vi "Untitled 1.vi"() -> ()   [LabVIEW 2023]
panel:
  in  "Saberi":bool
  in  "stop 2":bool
  in  "Podijeli":bool
  in  "Pomnozi":bool
  in  "Oduzmi":bool
  in  "Broj 2":dbl
  in  "Broj 1":dbl
  out "Rezultat":dbl
  in  "Pokreni":bool
  in  "Signal":enum16{"SINE", "COSINE"}(ring)
  out "Graph":dbl[](graph)
  out "XY Graph":cluster{dbl[], dbl[]}(graph)
  out "Waveform Graph 3":i32[](graph)
  out "Waveform Chart":i32[](graph)
  out "Waveform Graph 2":dynamicdata(graph)
  out "Waveform Graph":dynamicdata(graph)
  in  "stop":bool
  out "LED2":bool
  out "LED1":bool
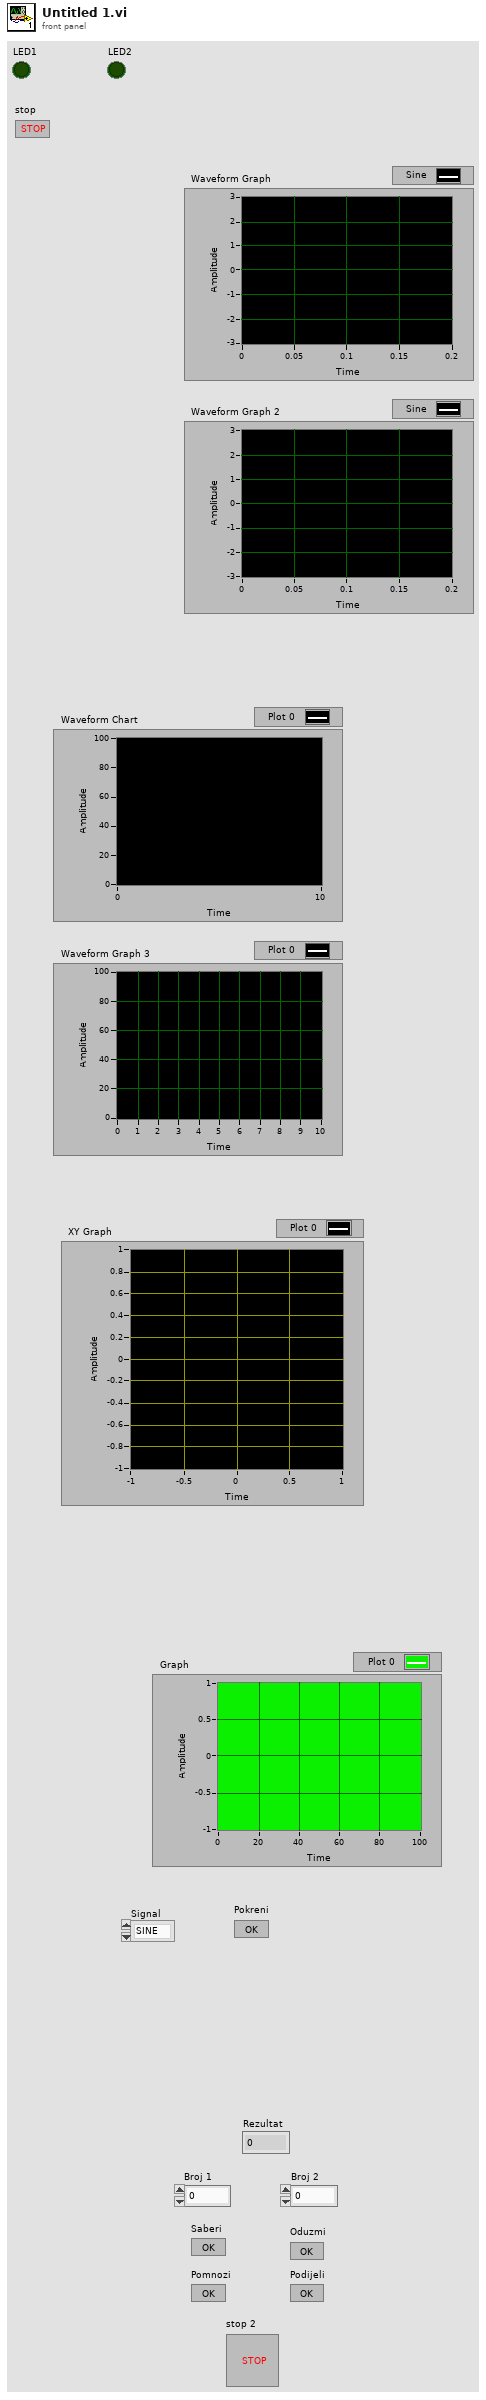
[diagram p1: front panel]
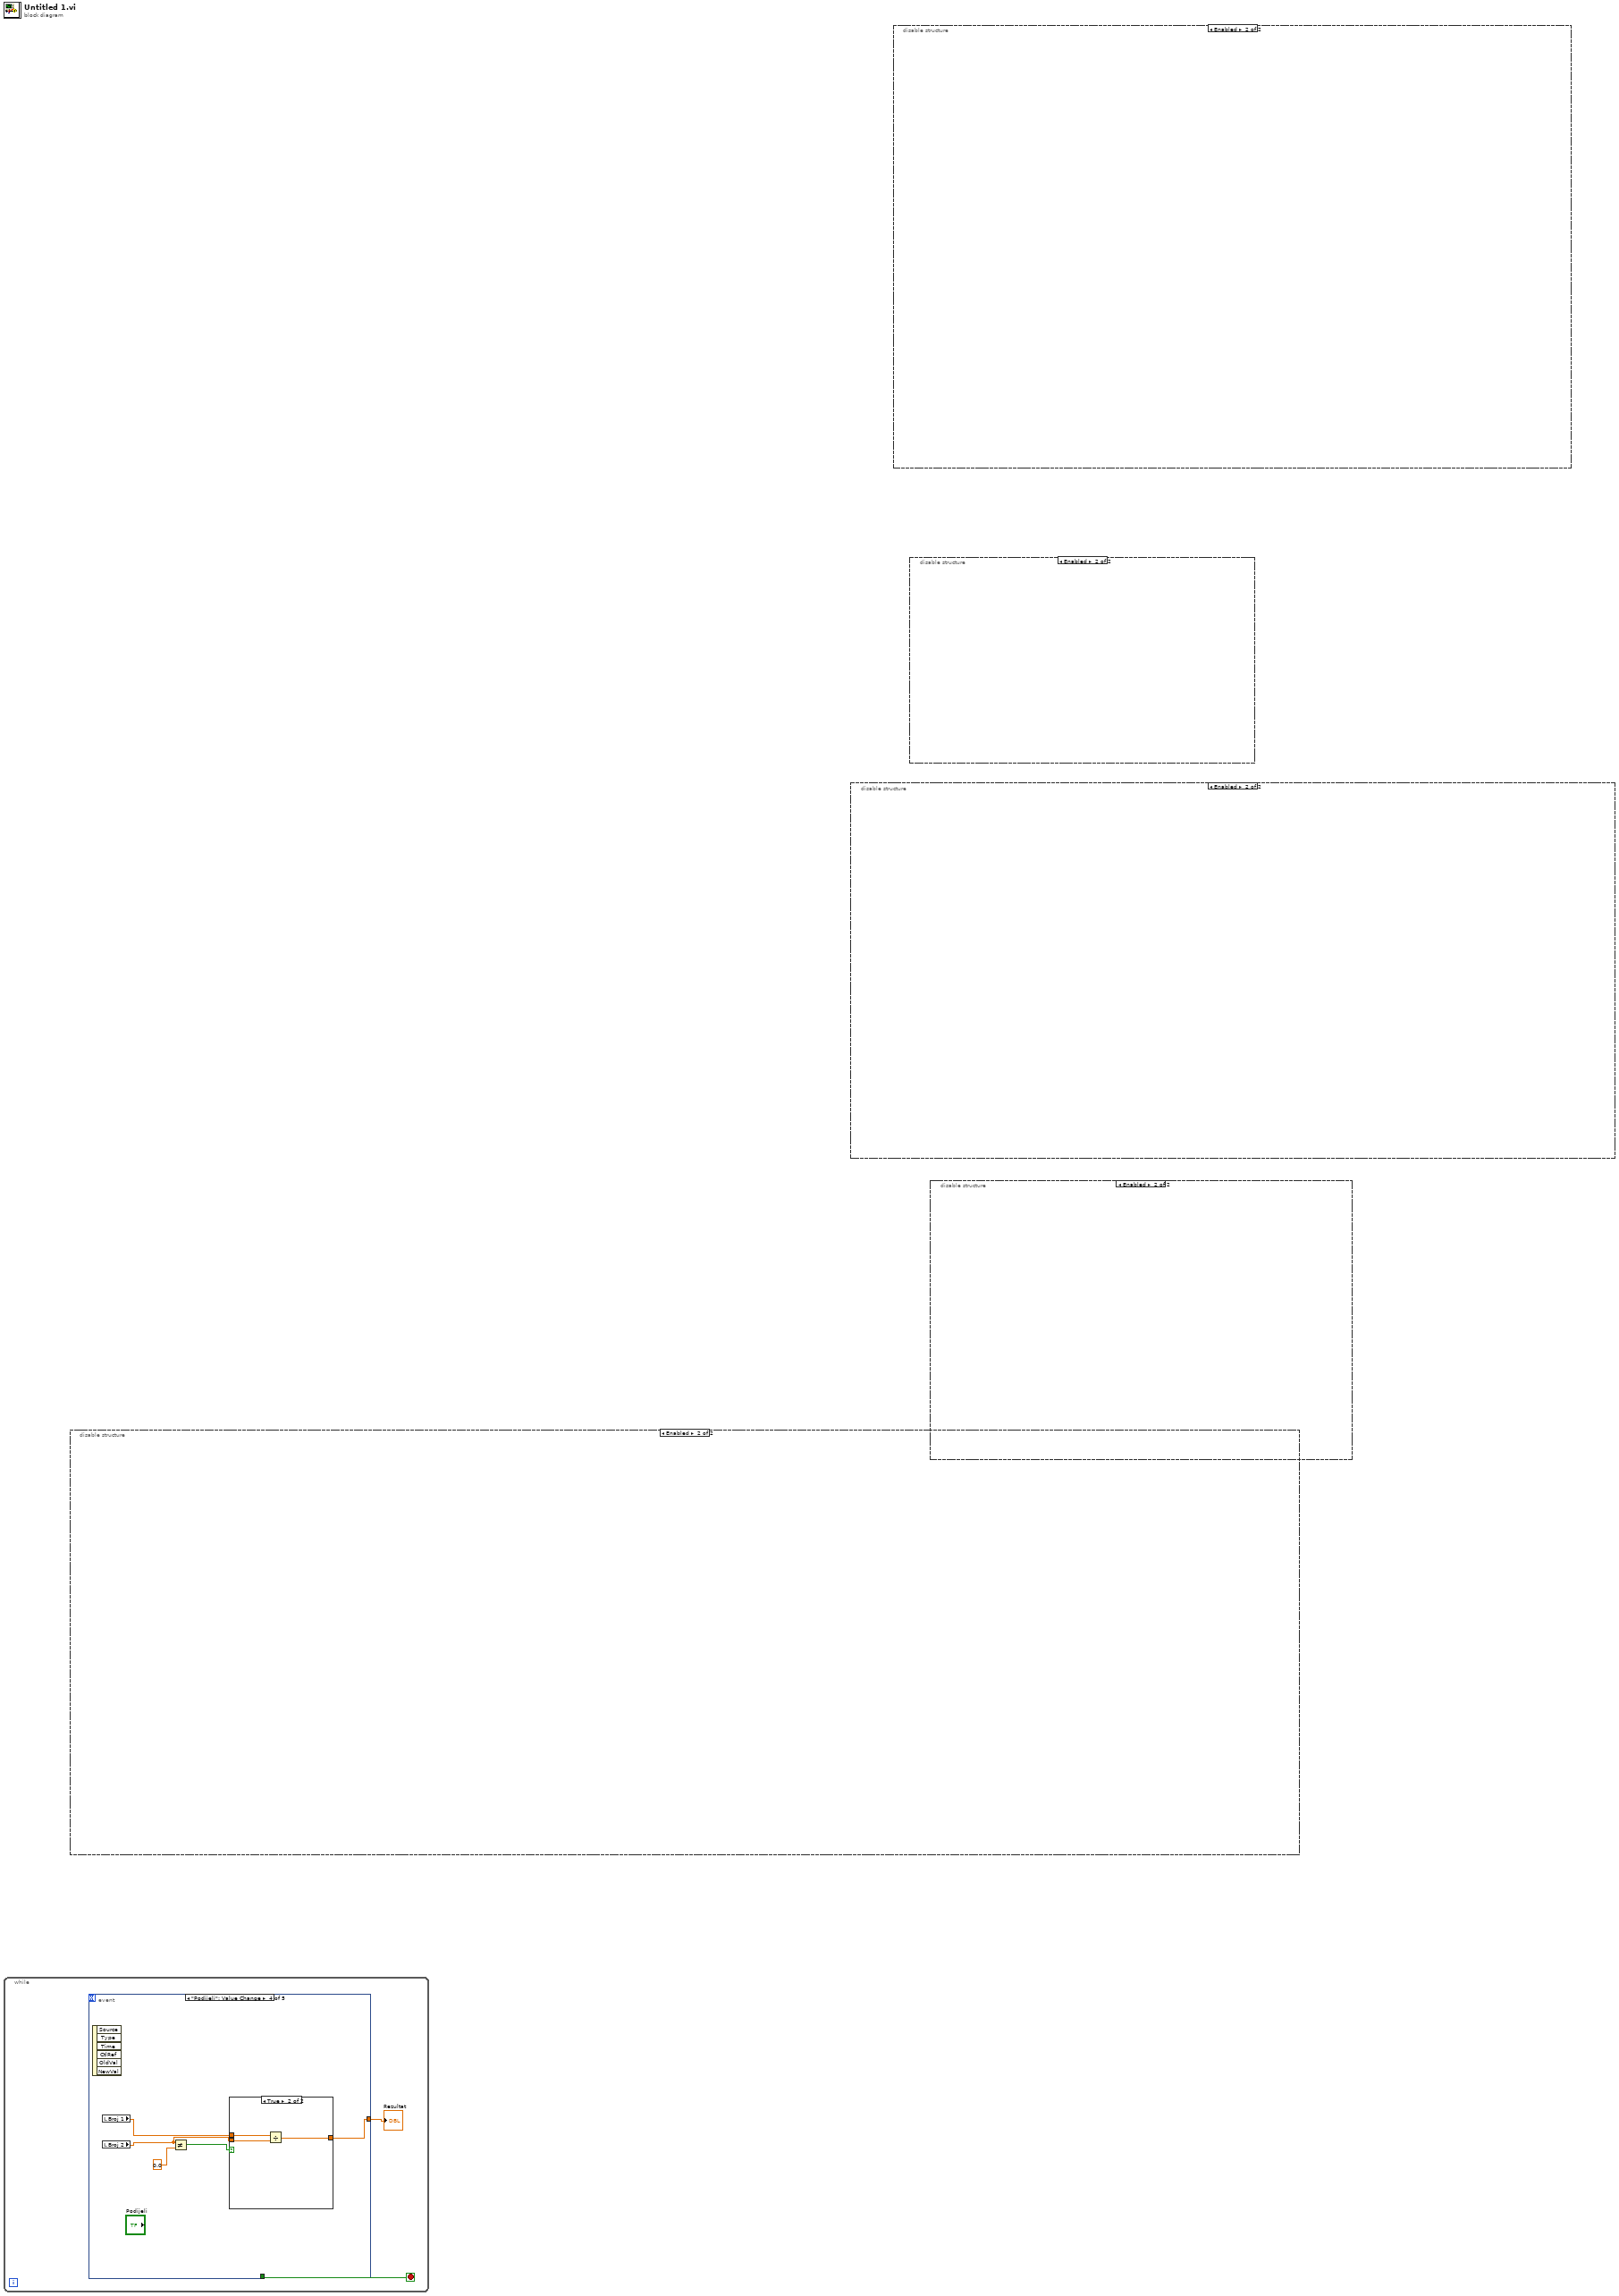
[diagram p0: block diagram]
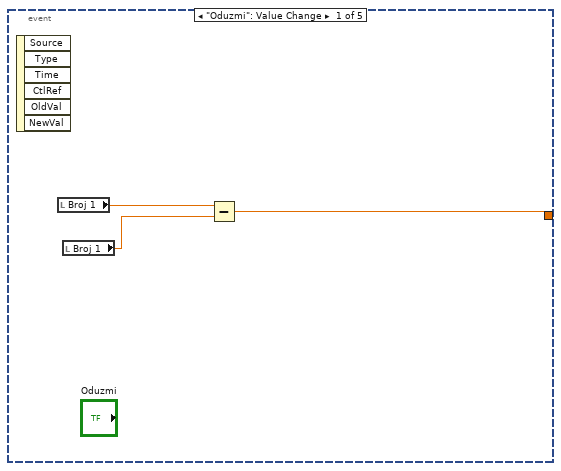
[diagram p2: hidden frame]
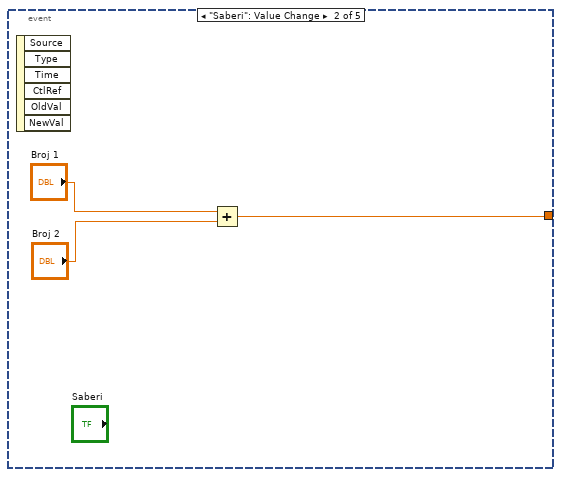
[diagram p3: hidden frame]
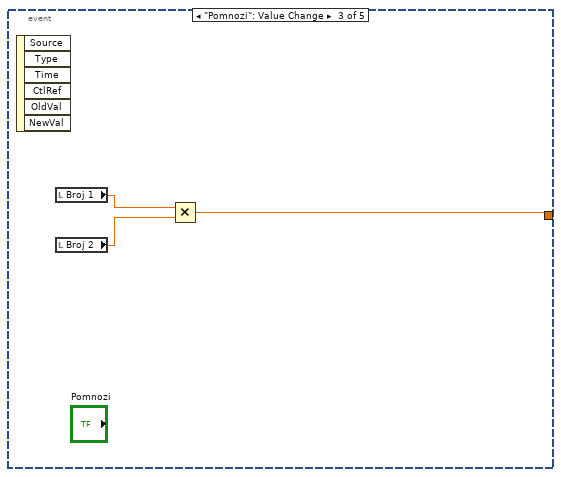
[diagram p4: hidden frame]
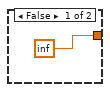
[diagram p5: hidden frame]
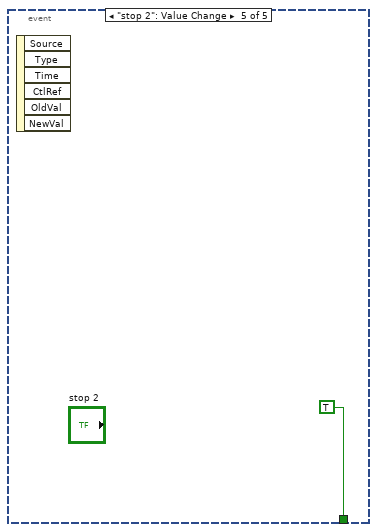
[diagram p6: hidden frame]
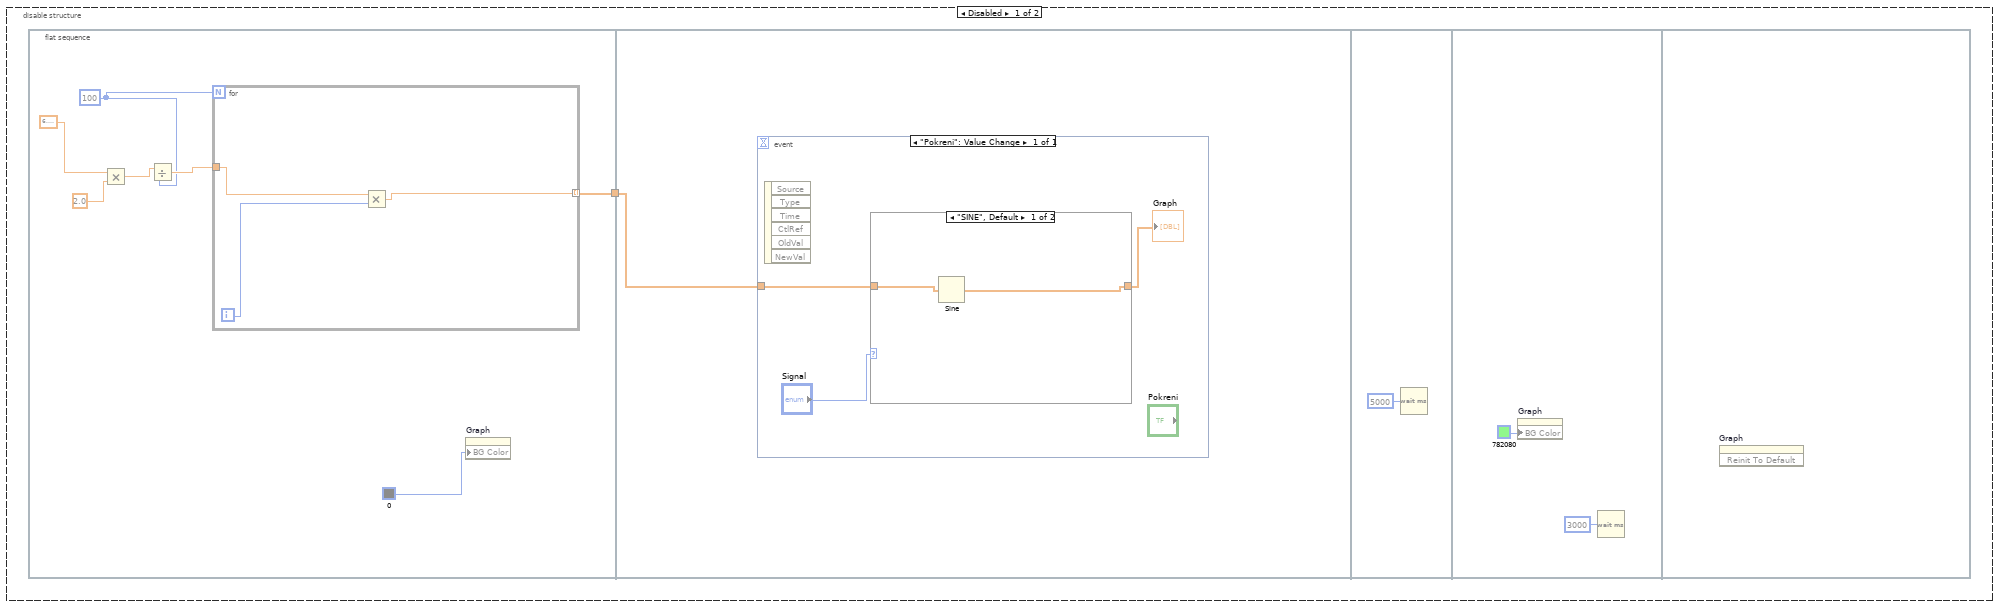
[diagram p7: hidden frame]
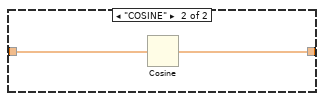
[diagram p8: hidden frame]
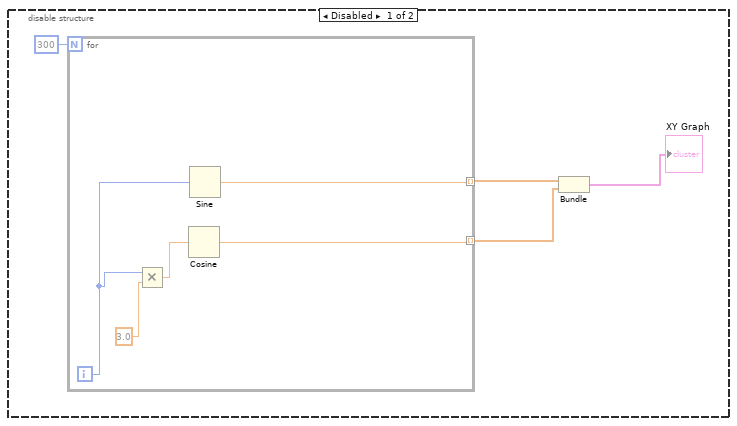
[diagram p9: hidden frame]
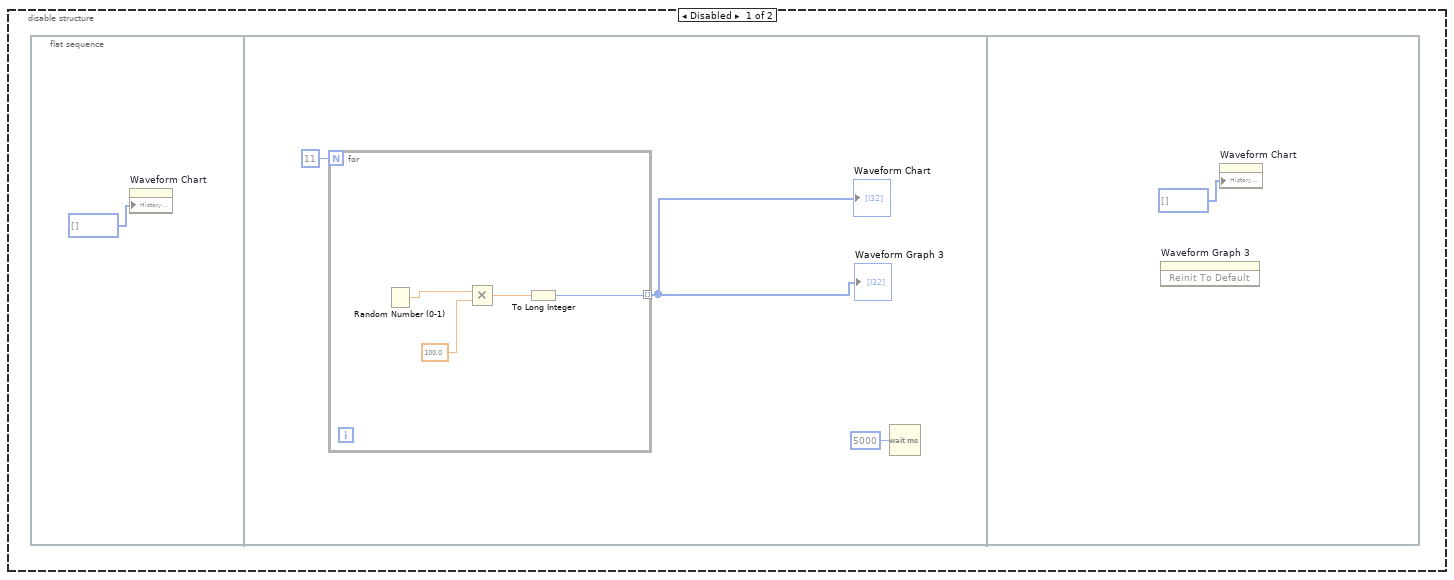
[diagram p10: hidden frame]
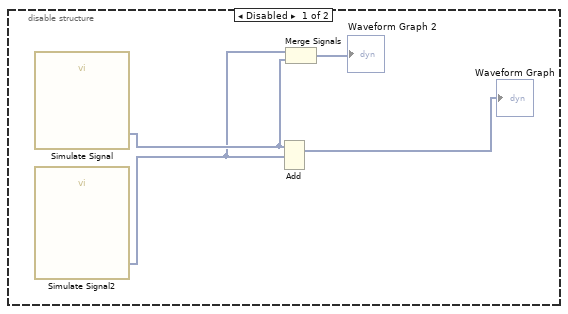
[diagram p11: hidden frame]
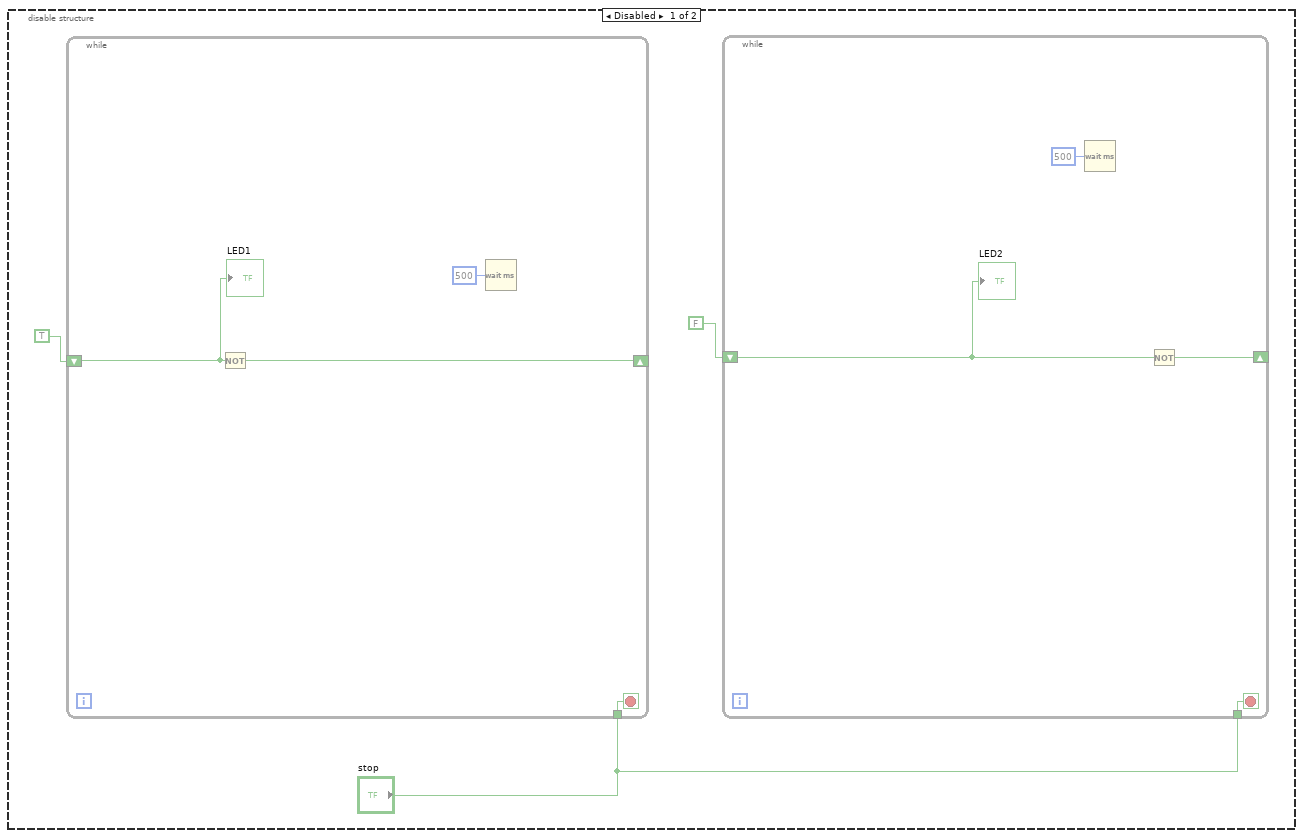
[diagram p12: hidden frame]
diagram:
  n1 = while {
    stop <- w2 stop-if-true
    n2 = event shown="[3] \"Podijeli\": Value Change" {
      selector: _ -> [_ _ _ _ _]
      dyn-events: _ -> [_ _ _ _ _]
      timeout: _ -> [_ _ _ _ _]
      tunnel: [w5 w8 w11 w14 _] -> w1
      tunnel: [_ _ _ _ TRUE] -> w2
      event "Oduzmi": Value Change {
        n3 = event-data() -> ()  [unwired: 1 in, 6 out]
        n4 = local read "Broj 1"() -> (w4:dbl)
        n5 = local read "Broj 1"() -> (w3:dbl)
        n6 = Subtract(x=w4, y=w3) -> (x-y=w5:dbl)
      }
      event "Saberi": Value Change {
        n7 = event-data() -> ()  [unwired: 1 in, 6 out]
        n8 = Add(x="Broj 1", y="Broj 2") -> (x+y=w8:dbl)
      }
      event "Pomnozi": Value Change {
        n9 = event-data() -> ()  [unwired: 1 in, 6 out]
        n10 = local read "Broj 1"() -> (w10:dbl)
        n11 = local read "Broj 2"() -> (w9:dbl)
        n12 = Multiply(x=w10, y=w9) -> (x*y=w11:dbl)
      }
      event "Podijeli": Value Change {
        n13 = event-data() -> ()  [unwired: 1 in, 6 out]
        n14 = local read "Broj 1"() -> (w13:dbl)
        n15 = local read "Broj 2"() -> (w12:dbl)
        n16 = Not Equal?(x=w12, y=0.0) -> (x != y?=w15:bool)
        n17 = case shown="True" w15 {
          tunnel: [inf w20] -> w14
          tunnel: w13 -> [_ w19]
          tunnel: w12 -> [_ w18]
          frame False {
          }
          frame True {
            n18 = Divide(x=w19, y=w18) -> (x/y=w20:dbl)
          }
        }
      }
      event "stop 2": Value Change {
        n19 = event-data() -> ()  [unwired: 1 in, 6 out]
      }
    }
    "Rezultat" <- w1
  }
  n20 = disable-structure shown="Enabled" {
    frame Disabled {
      n21 = flat-sequence {
        tunnel: [w24] -> w22
        tunnel: w22 -> [w33]
        frame #0 {
          w25 = 100
          n22 = Multiply(x=6.283185307179586, y=2.0) -> (x*y=w29:dbl)
          n23 = Divide(x=w29, y=w25) -> (x/y=w28:dbl)
          n24 = for {
            N: w25 -> [_]
            tunnel: w28 -> [w32]
            tunnel: [w30] -> w24 mode=indexing
            i -> [w31]
            n25 = Multiply(x=w32, y=w31) -> (x*y=w30:dbl)
          }
          n26 = property on="Graph" class="WFGraph (strict)"("BG Color"=u32 0 ("Plot Area:Colors:BG Color")) -> ()  [unwired: 2 in, 2 out]
        }
        frame #1 {
          n27 = event shown="[0] \"Pokreni\": Value Change" {
            selector: _ -> [_]
            dyn-events: _ -> [_]
            timeout: _ -> [_]
            tunnel: w33 -> [w35]
            event "Pokreni": Value Change {
              n28 = event-data() -> ()  [unwired: 1 in, 6 out]
              n29 = case shown="\"SINE\", Default" "Signal" {
                tunnel: [w38 w40] -> w34
                tunnel: w35 -> [w37 w39]
                frame "SINE", Default {
                  n30 = Sine(x=w37) -> (sin(x)=w38:dbl[])
                }
                frame "COSINE" {
                  n31 = Cosine(x=w39) -> (cos(x)=w40:dbl[])
                }
              }
              "Graph" <- w34
            }
          }
        }
        frame #2 {
          n32 = Wait (ms)(milliseconds to wait=u32 5000) -> ()  [unwired: 1 out]
        }
        frame #3 {
          n33 = property on="Graph" class="WFGraph (strict)"("BG Color"=u32 782080 ("Plot Area:Colors:BG Color")) -> ()  [unwired: 2 in, 2 out]
          n34 = Wait (ms)(milliseconds to wait=u32 3000) -> ()  [unwired: 1 out]
        }
        frame #4 {
          n35 = invoke on="Graph" class="WFGraph (strict)" method="Reinit To Default"() -> ()  [unwired: 3 in, 3 out]
        }
      }
    }
    frame Enabled {
    }
  }
  n36 = disable-structure shown="Enabled" {
    frame Disabled {
      n37 = flat-sequence {
        frame #0 {
          n38 = property on="Waveform Chart" class="WFChart (strict)"("History Data"=i32[] []) -> ()  [unwired: 2 in, 2 out]
        }
        frame #1 {
          n39 = for {
            N: 11 -> [_]
            tunnel: [w48] -> w46 mode=indexing
            n40 = Random Number (0-1)() -> (number: 0 to 1=w51:dbl)
            n41 = Multiply(x=w51, y=100.0) -> (x*y=w49:dbl)
            n42 = To Long Integer(number=w49) -> (32bit integer=w48:i32)
          }
          "Waveform Chart" <- w46
          "Waveform Graph 3" <- w46
          n43 = Wait (ms)(milliseconds to wait=u32 5000) -> ()  [unwired: 1 out]
        }
        frame #2 {
          n44 = invoke on="Waveform Graph 3" class="WFGraph (strict)" method="Reinit To Default"() -> ()  [unwired: 3 in, 3 out]
          n45 = property on="Waveform Chart" class="WFChart (strict)"("History Data"=i32[] []) -> ()  [unwired: 2 in, 2 out]
        }
      }
    }
    frame Enabled {
    }
  }
  n46 = disable-structure shown="Enabled" {
    frame Disabled {
      n47 = while {
        shift-right: [w62] -> _
        shift-left: TRUE -> [w61]
        tunnel: "stop" -> [w60]
        stop <- w60 stop-if-true
        n48 = Not(x=w61) -> (.not. x?=w62:bool)
        n49 = Wait (ms)(milliseconds to wait=u32 500) -> ()  [unwired: 1 out]
        "LED1" <- w61
      }
      n50 = while {
        shift-right: [w58] -> _
        shift-left: FALSE -> [w57]
        tunnel: "stop" -> [w56]
        stop <- w56 stop-if-true
        n51 = Wait (ms)(milliseconds to wait=u32 500) -> ()  [unwired: 1 out]
        n52 = Not(x=w57) -> (.not. x?=w58:bool)
        "LED2" <- w57
      }
    }
    frame Enabled {
    }
  }
  n53 = disable-structure shown="Enabled" {
    frame Disabled {
      n54 = call "Simulate Signal"() -> ("Sine"=w65:dynamicdata)  [unwired: 14 in, 1 out]
      n55 = call "Simulate Signal2"() -> ("Sine"=w64:dynamicdata)  [unwired: 14 in, 1 out]
      n56 = Add(1:w64, 2:w65) -> (0:→"Waveform Graph":dynamicdata)  [unwired: 1 in, 1 out]
      n57 = Merge Signals(w64, w65) -> (→"Waveform Graph 2":dynamicdata)
    }
    frame Enabled {
    }
  }
  n58 = disable-structure shown="Enabled" {
    frame Disabled {
      n59 = for {
        N: 300 -> [_]
        tunnel: [w73] -> w70 mode=indexing
        tunnel: [w72] -> w69 mode=indexing
        i -> [w75]
        n60 = Multiply(x=w75, y=3.0) -> (x*y=w74:dbl)
        n61 = Cosine(x=w74) -> (cos(x)=w72:dbl)
        n62 = Sine(x=w75) -> (sin(x)=w73:dbl)
      }
      n63 = Bundle(w70, w69) -> (→"XY Graph":cluster{dbl[], dbl[]})  [unwired: 1 in]
    }
    frame Enabled {
    }
  }
